vi "Mother_Segmenter.vi"(2 "Threshold Percentage":dbl, 3 "FFT Size":i32, 4 "Array in":dbl[](array[numeric])) -> (0 "Detected Wave":string, 1 "Dominant Frequency\nin Wave (Hz)":dbl)   [LabVIEW 2023]
panel:
  in  "Tab Control":T1(tab)
  out "Waveform Graph":cluster{i32, dbl, dbl[]}(graph)
  out "FFT Waveform Graph":dbl[](graph)
  out "Power Spectrum Graph":cluster{"f0":dbl, "df":dbl, "magnitude":dbl[]}(graph)
  out "abs(FFT) Waveform Graph":dbl[](graph)
  out "abs(FFT) Half Waveform Graph":dbl[](graph)
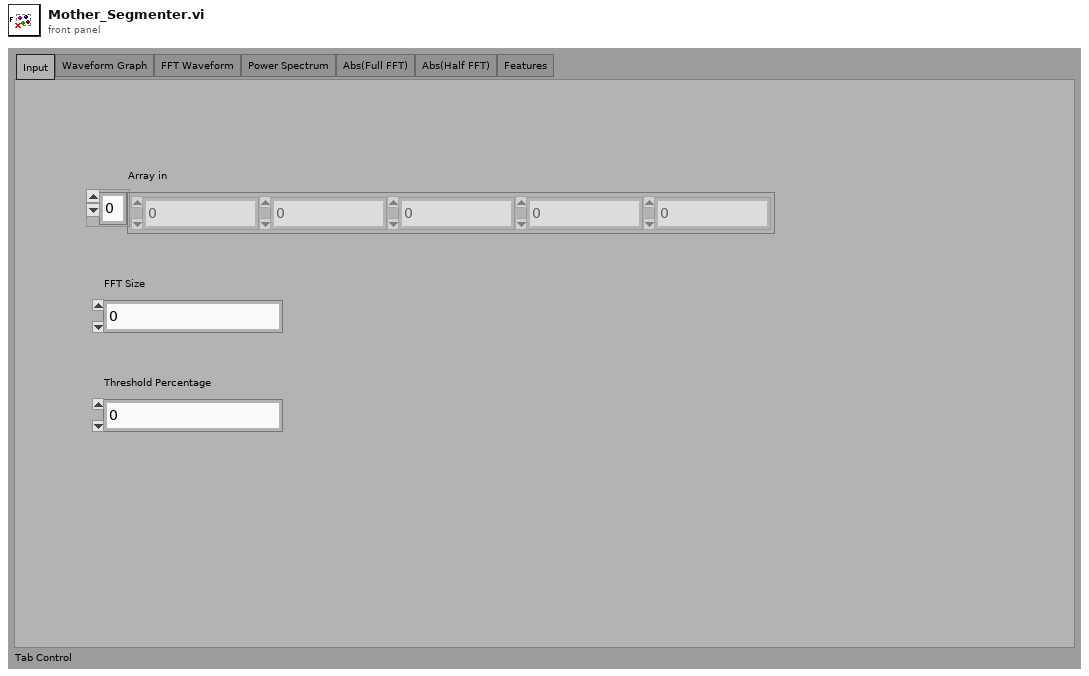
[diagram p1: front panel]
types:
  T1 = enum32{"Input", "Waveform Graph", "FFT Waveform", "Power Spectrum", "Abs(Full FFT)", "Abs(Half FFT)", "Features"}
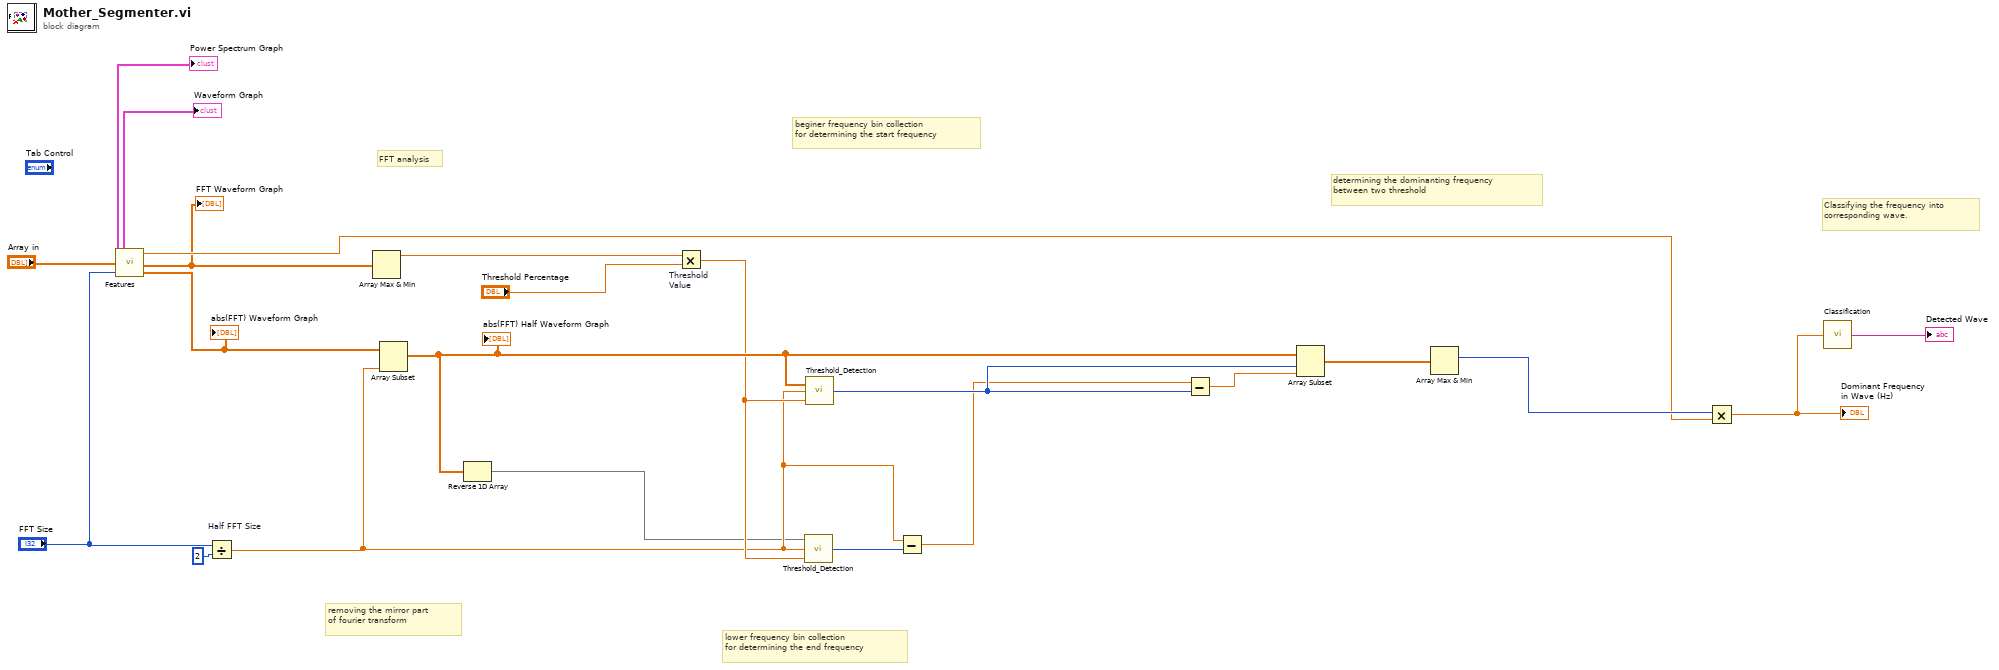
[diagram p0: block diagram]
diagram:
  # "FFT analysis"
  # "Classifying the frequency into\ncorresponding wave."
  # "determining the dominanting frequency\nbetween two threshold"
  # "beginer frequency bin collection\nfor determining the start frequency"
  # "lower frequency bin collection\nfor determining the end frequency"
  # "removing the mirror part\nof fourier transform"
  n1 = call "Features.vi"("Array in"="Array in", "Sampling"="FFT Size") -> ("Power Spectrum Graph"=→"Power Spectrum Graph":cluster{"f0":dbl, "df":dbl, "magnitude":dbl[]}, "Waveform Graph"=→"Waveform Graph":cluster{i32, dbl, dbl[]}, "Frequency Resolution"=w20:dbl, "FFT"=w3:dbl[], "abs(FFT)"=w5:dbl[])  [unwired: 2 in, 1 out]
  "FFT Waveform Graph" <- w3
  "abs(FFT) Waveform Graph" <- w5
  n2 = Divide "Half FFT Size"(x="FFT Size", y=2) -> (x/y=w12:dbl)
  n3 = Array Max & Min(array=w3) -> (max value=w9:dbl)  [unwired: 3 out]
  n4 = Array Subset "Array Subset"(array=w5, length=w12) -> (w15:dbl[])  [unwired: 1 in]
  "abs(FFT) Half Waveform Graph" <- w15
  n5 = Reverse 1D Array(array=w15) -> (reversed array=w10:dbl[])
  n6 = Multiply "Threshold\nValue"(x=w9, y="Threshold Percentage") -> (x*y=w13:dbl)
  n7 = call "Threshold_Detection.vi"("Threshold Value"=w13, "Length of Array"=w12, "Array"=w10) -> ("Detection Index"=w11:i32)
  n8 = call "Threshold_Detection.vi"("Threshold Value"=w13, "Length of Array"=w12, "Array"=w15) -> ("Detection Index"=w18:i32)
  n9 = Subtract(x=w12, y=w11) -> (x-y=w17:dbl)
  n10 = Subtract(x=w17, y=w18) -> (x-y=w16:dbl)
  n11 = Array Subset "Array Subset"(array=w15, index=w18, length=w16) -> (w19:dbl[])
  n12 = Array Max & Min(array=w19) -> (max index (indices)=w21:i32)  [unwired: 3 out]
  n13 = Multiply(x=w21, y=w20) -> (x*y=w4:dbl)
  "Dominant Frequency\nin Wave (Hz)" <- w4
  n14 = call "Classification.vi"("Numeric"=w4) -> ("Detected Wave"=→"Detected Wave":string)
